vi "Read Array Control.vi"(5 "section":string, 7 "Prefix":string, 8 "Error In":errorcluster, 10 "File refnum":T1, 11 "Ctl Refnum":refnum<vi>) -> (0 "Error Out":errorcluster, 2 "File refnum out":T1, 3 "Ctl Refnum out":refnum<vi>)   [LabVIEW 2015]
uses:
  <vilib>/Utility/config.llb/NI_LVConfig.lvlib
  <vilib>/Utility/config.llb/Read Key (I32).vi
  <vilib>/Utility/Data Type/NI_Data Type.lvlib
  <vilib>/Utility/config.llb/Config Data RefNum.ctl
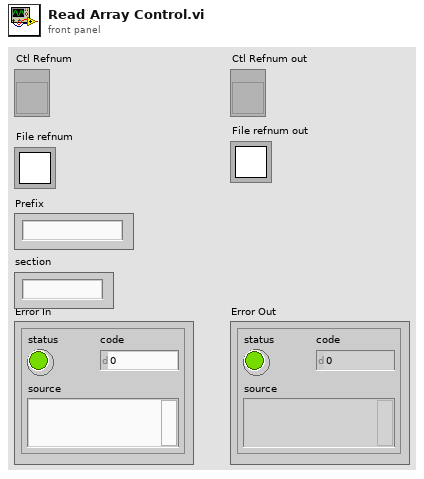
[diagram p1: front panel]
types:
  T1 = typedef "NI_LVConfig.lvlib/Config Data RefNum.ctl" = refnum<k1>
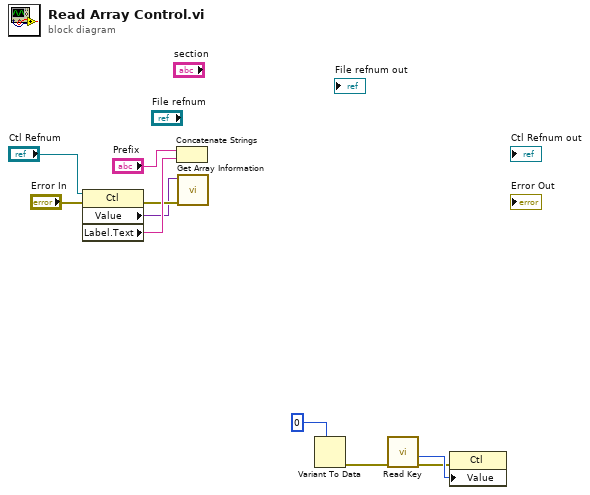
[diagram p0: block diagram]
diagram:
  n1 = property class="Ctl"(reference="Ctl Refnum", error in="Error In") -> (error out=w15:errorcluster, "Value"=w11:variant, "Label.Text"=w16:string)  [unwired: 1 out]
  n2 = Concatenate Strings("Prefix", w16) -> ()  [unwired: 1 out]
  n3 = call <vilib>:"Get Array Information.vi"("error in (no error)"=w15, "Variant"=w11) -> ()  [unwired: 6 in, 4 out]
  n4 = Variant To Data(type=0) -> (error in=w8:errorcluster, Variant=w10:i32, error out=w9:errorcluster)  [unwired: 1 out]
  n5 = call-poly <vilib>:"Read Key.vi"("error in (no error)"=w9) -> ("error out"=w5:errorcluster, "value"=w6:i32, "section"=w2:string, "key"=w3:string, "refnum"=w1:T1)  [unwired: 4 in, 2 out]
  n6 = property class="Ctl"(error in=w5, "Value"=w6) -> (reference=w4:refnum<vi>)  [unwired: 2 out]
